vi "set_pixel_times.vi"(8 "error in (no error)":errorcluster, 10 "pixel dwell time":dbl[unit], 11 "TrajectoryMG100122AODFrameScan in":refnum<class "TrajectoryMG100122AODFrameScan.lvclass">) -> (0 "error out":errorcluster, 3 "TrajectoryMG100122AODFrameScan out":refnum<class "TrajectoryMG100122AODFrameScan.lvclass">)   [LabVIEW 2010, in "TrajectoryMG100122AODFrameScan.lvclass"]
uses:
  TrajectoryMG100122AODFrameScan.lvclass
  TrajectoryMG100122AODFrameScan.lvclass/TrajectoryMG100122AODFrameScan.ctl
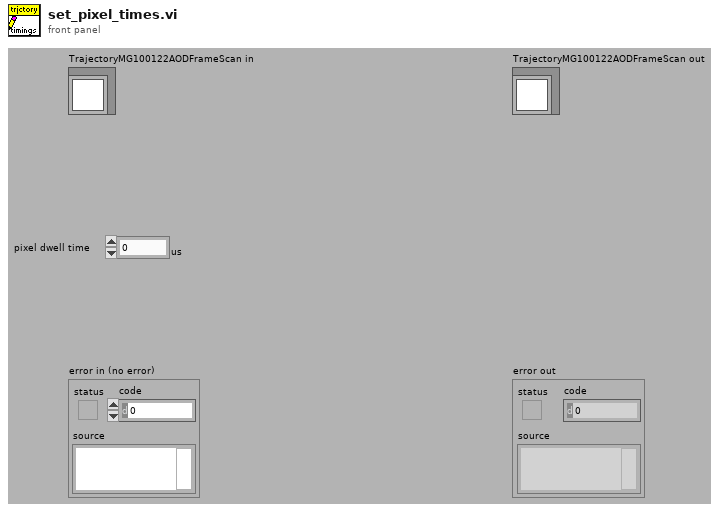
[diagram p1: front panel]
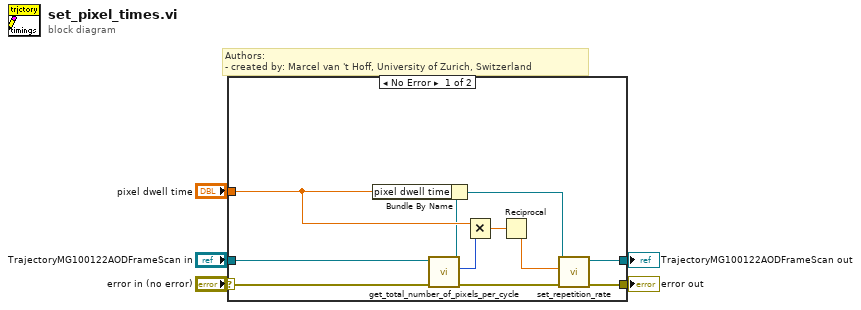
[diagram p0: block diagram]
diagram:
  # "Authors: \n- created by: Marcel van 't Hoff, University of Zurich, Switzerland"
  n1 = case shown="No Error" "error in (no error)" {
    selector: "error in (no error)" -> [w13 w17]
    tunnel: [w15 w17] -> w4
    tunnel: [w16 w18] -> w2
    tunnel: "TrajectoryMG100122AODFrameScan in" -> [w8 w18]
    tunnel: "pixel dwell time" -> [w10 _]
    frame No Error {
      n2 = call-dynamic "get_total_number_of_pixels_per_cycle.vi"("error in (no error)"=w13, "TrajectoryMG100122AODFrameScan in"=w8) -> ("error out"=w12:errorcluster, "total number of pixels per cycle"=w11:i32, "TrajectoryMG100122AODFrameScan out"=w7:refnum<class "TrajectoryMG100122AODFrameScan.lvclass">)  [unwired: 7 in]
      n3 = Bundle By Name(cluster=w7, "pixel dwell time"=w10) -> (w6:refnum<class "TrajectoryMG100122AODFrameScan.lvclass">)
      n4 = Multiply(x=w10, y=w11) -> (x*y=w9:dbl[unit])
      n5 = Reciprocal(x=w9) -> (1/x=w14:dbl[unit])
      n6 = call-dynamic "set_repetition_rate.vi"("error in (no error)"=w12, "repetition rate"=w14, "GenericTrajectory in"=w6) -> ("error out"=w15:errorcluster, "GenericTrajectory out"=w16:refnum<class "TrajectoryMG100122AODFrameScan.lvclass">)  [unwired: 7 in]
    }
    frame Error {
    }
  }
  "error out" <- w4
  "TrajectoryMG100122AODFrameScan out" <- w2
